vi "Encode Broadcast CAN-ID.vi"(10 "COB Broadcast":u16(ring) items=["NMT", "SYNC", "TIME"], 11 "Node ID":u8) -> (3 "CAN-ID":u16 format="%.0x")   [LabVIEW 2024, in "CANopen.lvlib" / "CANopen.lvclass"]
doc: "Computes the canonical COB-ID given the function code and the node ID. The implementation follows the algorithm described in CiA draft standard 301, page 78."
uses:
  CANopen.lvclass
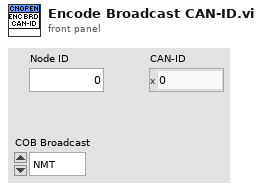
[diagram p1: front panel]
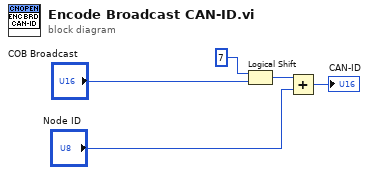
[diagram p0: block diagram]
diagram:
  n1 = Logical Shift(y=i16 7, x="COB Broadcast") -> (x << y=w4:u16)
  n2 = Add(x=w4, y="Node ID") -> (x+y=→"CAN-ID":u16)
